vi "lateral_and_vertical_acc.vi"(4 "Aerodyn output":T3, 5 "Vehicle Param":T2, 6 "Pdyn2":T1, 7 "FE_b [N], FG [N], FA [N], Fco[N]":T4, 8 "Data":dbl[][](array[numeric]), 9 "Time":T5, 10 "acc [m/s^2]":dbl[](array[numeric]), 11 "Rotation":T6) -> (3 "k_acc":cluster{"lat_acc_mod":dbl, "up_acc":dbl})   [LabVIEW 2017]
uses:
  <vilib>/Analysis/coordinate.llb/Euler Rotation Order.ctl
  <vilib>/Analysis/_algsub.llb/Vector Norm Type.ctl
  <vilib>/Analysis/_algsub.llb/Real Vector Norm.vi
  <vilib>/Analysis/baseanly.llb/Real A x B.vi
  <vilib>/Analysis/baseanly.llb/Real Dot Product.vi
  <vilib>/Analysis/Matrix/Numeric/Conversions/Array To Matrix - RA2.vi
  <vilib>/Analysis/Matrix/Numeric/Conversions/Matrix To Array - RM.vi
  <vilib>/Analysis/Matrix/Numeric/Conversions/Array To Matrix - RA.vi
  <vilib>/Analysis/NI_AALPro.lvlib
  <vilib>/Analysis/Matrix/NI_Matrix.lvlib
  <vilib>/Analysis/NI_AALBase.lvlib
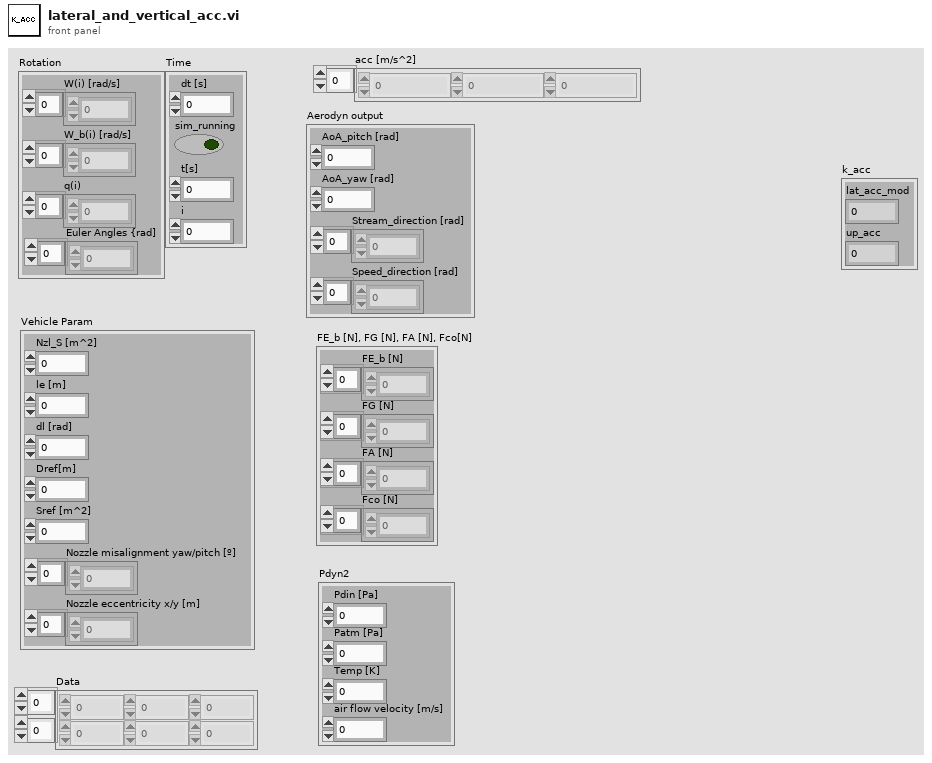
[diagram p1: front panel]
types:
  T1 = cluster{"Pdin [Pa]":dbl, "Patm [Pa]":dbl, "Temp [K]":dbl, "air flow velocity [m/s]":dbl}
  T2 = cluster{"Nzl_S [m^2]":dbl, "le [m]":dbl, "dl [rad]":dbl, "Dref[m]":dbl, "Sref [m^2]":dbl, "Nozzle misalignment yaw/pitch [º]":dbl[], "Nozzle eccentricity x/y [m]":dbl[]}
  T3 = cluster{"AoA_pitch [rad]":dbl, "AoA_yaw [rad]":dbl, "Stream_direction [rad]":dbl[], "Speed_direction [rad]":dbl[]}
  T4 = cluster{"FE_b [N]":dbl[], "FG [N]":dbl[], "FA [N]":dbl[], "Fco [N]":dbl[]}
  T5 = cluster{"dt [s]":dbl, "sim_running":bool, "t[s]":dbl, "i":i32}
  T6 = cluster{"W(i) [rad/s]":dbl[], "W_b(i) [rad/s]":dbl[], "q(i)":dbl[], "Euler Angles {rad]":dbl[]}
  T7 = typedef "NI_AALPro.lvlib/Vector Norm Type.ctl" = u16
  T8 = cluster{"AoA_pitch [rad]":dbl, "AoA_yaw [rad]":dbl, "Stream_direction [rad]":dbl[]}
  T9 = typedef "NI_AALPro.lvlib/Euler Rotation Order.ctl" = u16
  T10 = typedef "NI_Matrix.lvlib/RealMatrix.ctl" = dbl[][]
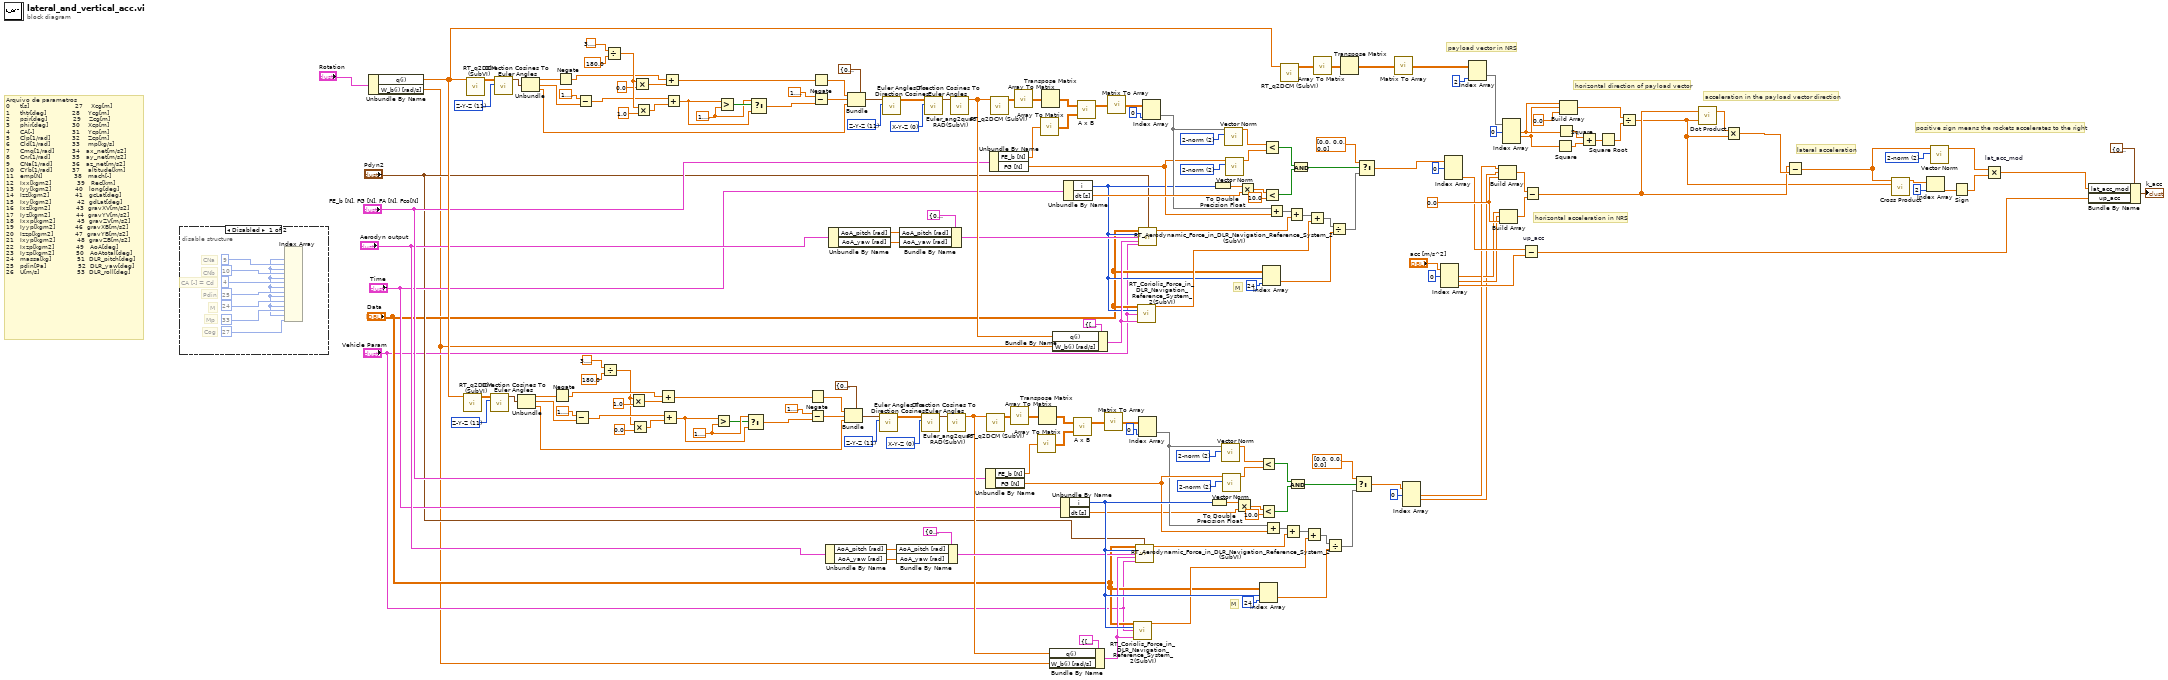
[diagram p0: block diagram]
diagram:
  w62 = T7 2 items=["1-norm"=1, "2-norm"=2, "Inf-norm"=3, "-Inf-norm"=4, "User Defined"=5] ("norm type")
  w61 = T7 2 items=["1-norm"=1, "2-norm"=2, "Inf-norm"=3, "-Inf-norm"=4, "User Defined"=5] ("norm type")
  w43 = T9 0 items=["X-Y-Z", "X-Z-Y", "Y-X-Z", "Y-Z-X", "Z-X-Y", "Z-Y-X", "X-Y-X", "X-Z-X", "Y-X-Y", "Y-Z-Y", "Z-X-Z", "Z-Y-Z"] ("rotation order")
  w42 = T9 11 items=["X-Y-Z", "X-Z-Y", "Y-X-Z", "Y-Z-X", "Z-X-Y", "Z-Y-X", "X-Y-X", "X-Z-X", "Y-X-Y", "Y-Z-Y", "Z-X-Z", "Z-Y-Z"] ("rotation order")
  w33 = 1.5707963267948966
  w17 = T9 11 items=["X-Y-Z", "X-Z-Y", "Y-X-Z", "Y-Z-X", "Z-X-Y", "Z-Y-X", "X-Y-X", "X-Z-X", "Y-X-Y", "Y-Z-Y", "Z-X-Z", "Z-Y-Z"] ("rotation order")
  w97 = T7 2 items=["1-norm"=1, "2-norm"=2, "Inf-norm"=3, "-Inf-norm"=4, "User Defined"=5] ("norm type")
  w113 = 0.0 ("element")
  w143 = T7 2 items=["1-norm"=1, "2-norm"=2, "Inf-norm"=3, "-Inf-norm"=4, "User Defined"=5] ("norm type")
  w144 = T7 2 items=["1-norm"=1, "2-norm"=2, "Inf-norm"=3, "-Inf-norm"=4, "User Defined"=5] ("norm type")
  w162 = T9 0 items=["X-Y-Z", "X-Z-Y", "Y-X-Z", "Y-Z-X", "Z-X-Y", "Z-Y-X", "X-Y-X", "X-Z-X", "Y-X-Y", "Y-Z-Y", "Z-X-Z", "Z-Y-Z"] ("rotation order")
  w163 = T9 11 items=["X-Y-Z", "X-Z-Y", "Y-X-Z", "Y-Z-X", "Z-X-Y", "Z-Y-X", "X-Y-X", "X-Z-X", "Y-X-Y", "Y-Z-Y", "Z-X-Z", "Z-Y-Z"] ("rotation order")
  w172 = 1.5707963267948966
  w188 = T9 11 items=["X-Y-Z", "X-Z-Y", "Y-X-Z", "Y-Z-X", "Z-X-Y", "Z-Y-X", "X-Y-X", "X-Z-X", "Y-X-Y", "Y-Z-Y", "Z-X-Z", "Z-Y-Z"] ("rotation order")
  # "M"
  # "positive sign means the rockets accelerates to the right"
  # "lateral acceleration"
  # "acceleration in the payload vector direction"
  # "horizontal direction of payload vector"
  # "horizontal acceleration in NRS"
  # "payload vector in NRS"
  # "M"
  # "Arquivo de parametros\n0     t[s]                       27    Xcg[m] \n1     thtr[deg]             28    Ycg[m]\n2     psir[deg]             29    Zcg[m]  \n3     phir[deg]            30    Xcp[m]       \n4     CA[-]                   31    Ycp[m]        \n5     Clp[1/rad]           32    Zcp[m]     \n6     Cld[1/rad]           33    mp[kg/s]        \n7     Cmq[1/rad]         34   ax_net[m/s2]         \n8     Cnr[1/rad]           35   ay_net[m/s2]      \n9     CNa[1/rad]          36   az_net[m/s2]      \n10   CYb[1/rad]          37    altitude[km]       \n11   emp[N]                38   mach[-]     \n12   Ixx[kgm2]             39   Rec[km]     \n13   Iyy[kgm2]            40   long[deg]     \n14   Izz[kgm2]             41   gcLat[deg]        \n15   Ixy[kgm2]             42  gdLat[deg]       \n16   Ixz[kgm2]             43  gravXV[m/s2]  \n17   Iyz[kgm2]             44  gravYV[m/s2]     \n18   Ixxp[kgm2]           45  gravZV[m/s2]         \n19   Iyyp[kgm2]          46  gravXB[m/s2]         \n20   Izzp[kgm2]           47  gravYB[m/s2]         \n21   Ixyp[kgm2]           48  gravZB[m/s2]           \n22   Ixzp[kgm2]           49   AoA[deg]             \n23   Iyzp[kgm2]           50   AoAtotal[deg]       \n24   massa[kg]             51  DLR_pitch[deg]    \n25   pdin[Pa]                52  DLR_yaw[deg]  \n26   U[m/s]                   53  DLR_roll[deg]"
  n1 = disable-structure shown="Disabled" {
    frame Disabled {
      # "Cog"
      # "Mp"
      # "M"
      # "Pdin"
      # "CA [-] = Cd"
      # "CNb"
      # "CNa"
      n2 = Index Array(index (col) #1=9 ("disabled index (col)"), index (row) #2=w191, index (col) #2=10 ("disabled index (col)"), index (row) #3=w191, index (col) #3=4 ("disabled index (col)"), index (row) #4=w191, index (col) #4=25 ("disabled index (col)"), index (row) #5=w191, index (col) #5=24 ("disabled index (col)"), index (row) #6=w191, index (col) #6=33 ("disabled index (col)"), index (row) #7=w191, index (col) #7=27 ("disabled index (col)")) -> (index (row) #1=w191:i32)  [unwired: 1 in, 7 out]
    }
    frame Enabled {
    }
  }
  n3 = Unbundle By Name("Rotation") -> ("q(i)"=w15:dbl[], "W_b(i) [rad/s]"=w8:dbl[])
  n4 = call "RT_q2DCM (SubVI).vi"("Quaternion"=w15) -> ("DCM"=w16:dbl[][])  [unwired: 10 in]
  n5 = call "RT_q2DCM (SubVI).vi"("Quaternion"=w15) -> ("DCM"=w189:dbl[][])  [unwired: 10 in]
  n6 = call <vilib>:"Direction Cosines To Euler Angles.vi"("rotation order"=w17, "Direction Cosines"=w16) -> ("Euler Angles"=w18:cluster{"phi":dbl, "theta":dbl, "psi":dbl})  [unwired: 8 in, 1 out]
  n7 = call <vilib>:"Direction Cosines To Euler Angles.vi"("rotation order"=w188, "Direction Cosines"=w189) -> ("Euler Angles"=w187:cluster{"phi":dbl, "theta":dbl, "psi":dbl})  [unwired: 8 in, 1 out]
  n8 = Unbundle(w18) -> ("phi"=w19:dbl, "theta"=w21:dbl, "psi"=w40:dbl)
  n9 = Unbundle(w187) -> ("phi"=w186:dbl, "theta"=w184:dbl, "psi"=w165:dbl)
  n10 = Negate(x=w19) -> (-x=w28:dbl)
  n11 = Negate(x=w186) -> (-x=w177:dbl)
  n12 = Subtract(x=1.5707963267948966, y=w21) -> (x-y=w30:dbl)
  n13 = Subtract(x=1.5707963267948966, y=w184) -> (x-y=w175:dbl)
  n14 = Divide(x=3.141592653589793, y=180.0) -> (x/y=w24:dbl)
  n15 = Divide(x=3.141592653589793, y=180.0) -> (x/y=w181:dbl)
  n16 = Multiply(x=w24, y=1.0) -> (x*y=w27:dbl)
  n17 = Multiply(x=w24, y=0.0) -> (x*y=w29:dbl)
  n18 = Multiply(x=w181, y=0.0) -> (x*y=w178:dbl)
  n19 = Multiply(x=w181, y=1.0) -> (x*y=w176:dbl)
  n20 = Add(x=w28, y=w27) -> (x+y=w35:dbl)
  n21 = Add(x=w30, y=w29) -> (x+y=w32:dbl)
  n22 = Add(x=w177, y=w178) -> (x+y=w170:dbl)
  n23 = Add(x=w175, y=w176) -> (x+y=w173:dbl)
  n24 = Greater?(x=w32, y=w33) -> (0:w31:bool)
  n25 = Greater?(x=w173, y=w172) -> (0:w174:bool)
  n26 = Select(t=w33, s=w31, f=w32) -> (s? t:f=w38:dbl)
  n27 = Select(t=w172, s=w174, f=w173) -> (s? t:f=w167:dbl)
  n28 = Negate(x=w35) -> (-x=w36:dbl)
  n29 = Subtract(x=1.5707963267948966, y=w38) -> (x-y=w39:dbl)
  n30 = Negate(x=w170) -> (-x=w169:dbl)
  n31 = Subtract(x=1.5707963267948966, y=w167) -> (x-y=w166:dbl)
  n32 = Unbundle By Name("Aerodyn output") -> ("AoA_pitch [rad]"=w58:dbl, "AoA_yaw [rad]"=w59:dbl)
  n33 = Unbundle By Name("Aerodyn output") -> ("AoA_pitch [rad]"=w147:dbl, "AoA_yaw [rad]"=w146:dbl)
  n34 = Bundle(cluster=cluster{"phi":dbl, "theta":dbl, "psi":dbl} {"phi"=0.0, "theta"=0.0, "psi"=0.0} ("Euler Angles"), "phi"=w36, "theta"=w39, "psi"=w40) -> (w41:cluster{"phi":dbl, "theta":dbl, "psi":dbl})
  n35 = Bundle(cluster=cluster{"phi":dbl, "theta":dbl, "psi":dbl} {"phi"=0.0, "theta"=0.0, "psi"=0.0} ("Euler Angles"), "phi"=w169, "theta"=w166, "psi"=w165) -> (w164:cluster{"phi":dbl, "theta":dbl, "psi":dbl})
  n36 = call <vilib>:"Euler Angles To Direction Cosines.vi"("rotation order"=w42, "Euler Angles"=w41) -> ("Direction Cosines"=w44:dbl[][])  [unwired: 8 in, 1 out]
  n37 = call <vilib>:"Euler Angles To Direction Cosines.vi"("rotation order"=w163, "Euler Angles"=w164) -> ("Direction Cosines"=w161:dbl[][])  [unwired: 8 in, 1 out]
  n38 = Bundle By Name(cluster=T8 {"AoA_pitch [rad]"=0.0, "AoA_yaw [rad]"=0.0, "Stream_direction [rad]"=[]} ("output cluster"), "AoA_pitch [rad]"=w58, "AoA_yaw [rad]"=w59) -> (w57:T8)
  n39 = Bundle By Name(cluster=T8 {"AoA_pitch [rad]"=0.0, "AoA_yaw [rad]"=0.0, "Stream_direction [rad]"=[]} ("output cluster"), "AoA_pitch [rad]"=w147, "AoA_yaw [rad]"=w146) -> (w148:T8)
  n40 = call <vilib>:"Direction Cosines To Euler Angles.vi"("rotation order"=w43, "Direction Cosines"=w44) -> ("Euler Angles"=w45:cluster{"phi":dbl, "theta":dbl, "psi":dbl})  [unwired: 8 in, 1 out]
  n41 = call <vilib>:"Direction Cosines To Euler Angles.vi"("rotation order"=w162, "Direction Cosines"=w161) -> ("Euler Angles"=w160:cluster{"phi":dbl, "theta":dbl, "psi":dbl})  [unwired: 8 in, 1 out]
  n42 = call "Euler_ang2quat RAD(SubVI).vi"("Euler Angles [rad]"=w45) -> ("Quaternions"=w55:dbl[])  [unwired: 10 in]
  n43 = call "Euler_ang2quat RAD(SubVI).vi"("Euler Angles [rad]"=w160) -> ("Quaternions"=w150:dbl[])  [unwired: 10 in]
  n44 = Unbundle By Name("FE_b [N], FG [N], FA [N], Fco[N]") -> ("FE_b [N]"=w50:dbl[], "FG [N]"=w76:dbl[])
  n45 = call "RT_q2DCM (SubVI).vi"("Quaternion"=w55) -> ("DCM"=w46:dbl[][])  [unwired: 10 in]
  n46 = Unbundle By Name("FE_b [N], FG [N], FA [N], Fco[N]") -> ("FE_b [N]"=w155:dbl[], "FG [N]"=w129:dbl[])
  n47 = call "RT_q2DCM (SubVI).vi"("Quaternion"=w150) -> ("DCM"=w159:dbl[][])  [unwired: 10 in]
  n48 = call-poly <vilib>:"Array To Matrix.vi"("Real 2D Array"=w46) -> ("Real Matrix"=w47:T10)
  n49 = call-poly <vilib>:"Array To Matrix.vi"("Real 2D Array"=w159) -> ("Real Matrix"=w158:T10)
  n50 = call-poly <vilib>:"Array To Matrix.vi"("Real 1D Array"=w50) -> ("Real Matrix (Column Vector)"=w49:T10)
  n51 = Transpose Matrix(1:w47) -> (0:w48:T10)
  n52 = call-poly <vilib>:"Array To Matrix.vi"("Real 1D Array"=w155) -> ("Real Matrix (Column Vector)"=w156:T10)
  n53 = Transpose Matrix(1:w158) -> (0:w157:T10)
  n54 = Bundle By Name(cluster=T6 {"W(i) [rad/s]"=[], "W_b(i) [rad/s]"=[], "q(i)"=[], "Euler Angles {rad]"=[]} ("Rotation 2"), "q(i)"=w55, "W_b(i) [rad/s]"=w8) -> (w60:T6)
  n55 = Bundle By Name(cluster=T6 {"W(i) [rad/s]"=[], "W_b(i) [rad/s]"=[], "q(i)"=[], "Euler Angles {rad]"=[]} ("Rotation 2"), "q(i)"=w150, "W_b(i) [rad/s]"=w8) -> (w145:T6)
  n56 = Unbundle By Name("Time") -> ("i"=w79:i32, "dt [s]"=w65:dbl)
  n57 = Unbundle By Name("Time") -> ("i"=w126:i32, "dt [s]"=w140:dbl)
  n58 = call-poly <vilib>:"A x B.vi"("B"=w49, "A"=w48) -> ("A x B"=w53:T10)  [unwired: 1 out]
  n59 = call-poly <vilib>:"A x B.vi"("B"=w156, "A"=w157) -> ("A x B"=w152:T10)  [unwired: 1 out]
  n60 = call-poly <vilib>:"Matrix To Array.vi"("Real Matrix"=w53) -> ("Real 2D Array"=w51:dbl[][])
  n61 = call-poly <vilib>:"Matrix To Array.vi"("Real Matrix"=w152) -> ("Real 2D Array"=w154:dbl[][])
  n62 = call "RT_Coriolis_Force_in_DLR_Navigation_Reference_System_2(SubVI).vi"("Data"="Data", "i"=w79, "Vehicle Parameters"="Vehicle Param", "Rotation"=w60) -> ("Fco (N)"=w78:dbl[])  [unwired: 11 in]
  n63 = call "RT_Aerodynamic_Force_in_DLR_Navigation_Reference_System_2 (SubVI).vi"("Data"="Data", "input cluster 3"="Pdyn2", "i"=w79, "output cluster"=w57, "Rotation"=w60, "Vehicle Parameters"="Vehicle Param") -> ("FA"=w77:dbl[])  [unwired: 8 in, 1 out]
  n64 = call "RT_Coriolis_Force_in_DLR_Navigation_Reference_System_2(SubVI).vi"("Data"="Data", "i"=w126, "Vehicle Parameters"="Vehicle Param", "Rotation"=w145) -> ("Fco (N)"=w127:dbl[])  [unwired: 11 in]
  n65 = call "RT_Aerodynamic_Force_in_DLR_Navigation_Reference_System_2 (SubVI).vi"("Data"="Data", "input cluster 3"="Pdyn2", "i"=w126, "output cluster"=w148, "Rotation"=w145, "Vehicle Parameters"="Vehicle Param") -> ("FA"=w128:dbl[])  [unwired: 8 in, 1 out]
  n66 = Index Array(array=w51, index (col)=0 ("index (row)")) -> (element=w75:dbl[])  [unwired: 1 in]
  n67 = Index Array(array=w154, index (col)=0 ("index (row)")) -> (element=w130:dbl[])  [unwired: 1 in]
  n68 = To Double Precision Float(number=w79) -> (double precision float=w66:dbl)
  n69 = To Double Precision Float(number=w126) -> (double precision float=w139:dbl)
  n70 = call-poly <vilib>:"Vector Norm.vi"("norm type"=w61, "Input Vector"=w75) -> ("norm"=w63:dbl)  [unwired: 8 in, 1 out]
  n71 = call-poly <vilib>:"Vector Norm.vi"("norm type"=w62, "Input Vector"=w76) -> ("norm"=w64:dbl)  [unwired: 8 in, 1 out]
  n72 = call-poly <vilib>:"Vector Norm.vi"("norm type"=w144, "Input Vector"=w130) -> ("norm"=w142:dbl)  [unwired: 8 in, 1 out]
  n73 = call-poly <vilib>:"Vector Norm.vi"("norm type"=w143, "Input Vector"=w129) -> ("norm"=w141:dbl)  [unwired: 8 in, 1 out]
  n74 = Multiply(x=w66, y=w65) -> (x*y=w67:dbl)
  n75 = Multiply(x=w139, y=w140) -> (x*y=w138:dbl)
  n76 = Index Array(array="Data", index (row)=w79, index (col)=24 ("disabled index (col)")) -> (element=w82:dbl)
  n77 = Less?(x=w63, y=w64) -> (x < y?=w69:bool)
  n78 = Less?(x=w67, y=10.0) -> (x < y?=w70:bool)
  n79 = Index Array(array="Data", index (row)=w126, index (col)=24 ("disabled index (col)")) -> (element=w123:dbl)
  n80 = Less?(x=w142, y=w141) -> (x < y?=w136:bool)
  n81 = Less?(x=w138, y=10.0) -> (x < y?=w135:bool)
  n82 = Add(x=w75, y=w76) -> (x+y=w73:dbl[])
  n83 = Add(x=w130, y=w129) -> (x+y=w132:dbl[])
  n84 = call "RT_q2DCM (SubVI).vi"("Quaternion"=w15) -> ("DCM"=w120:dbl[][])  [unwired: 10 in]
  n85 = Add(x=w73, y=w77) -> (x+y=w74:dbl[])
  n86 = Add(x=w132, y=w128) -> (x+y=w131:dbl[])
  n87 = And(x=w69, y=w70) -> (x .and. y?=w71:bool)
  n88 = And(x=w136, y=w135) -> (x .and. y?=w134:bool)
  n89 = Add(x=w74, y=w78) -> (x+y=w81:dbl[])
  n90 = Add(x=w131, y=w127) -> (x+y=w124:dbl[])
  n91 = call-poly <vilib>:"Array To Matrix.vi"("Real 2D Array"=w120) -> ("Real Matrix"=w121:T10)
  n92 = Divide(x=w81, y=w82) -> (x/y=w83:dbl[])
  n93 = Divide(x=w124, y=w123) -> (x/y=w122:dbl[])
  n94 = Transpose Matrix(1:w121) -> (0:w117:T10)
  n95 = Select(t=dbl[] [0.0, 0.0, 0.0], s=w71, f=w83) -> (s? t:f=w2:dbl[])
  n96 = Select(t=dbl[] [0.0, 0.0, 0.0], s=w134, f=w122) -> (s? t:f=w84:dbl[])
  n97 = call-poly <vilib>:"Matrix To Array.vi"("Real Matrix"=w117) -> ("Real 2D Array"=w118:dbl[][])
  n98 = Index Array(array=w2, index #1=0 ("index")) -> (element #1=w6:dbl, element #2=w3:dbl)  [unwired: 2 in, 1 out]
  n99 = Index Array(array="acc [m/s^2]", index #1=0 ("index")) -> (element #1=w5:dbl, element #2=w4:dbl, element #3=w89:dbl)  [unwired: 2 in]
  n100 = Index Array(array=w84, index #1=0 ("index")) -> (element #3=w90:dbl)  [unwired: 2 in, 2 out]
  n101 = Index Array(array=w118, index (col)=2 ("index (row)")) -> (element=w109:dbl[])  [unwired: 1 in]
  n102 = Build Array(w6, w3, w113) -> (w112:dbl[])
  n103 = Build Array(w5, w4, w113) -> (w111:dbl[])
  n104 = Index Array(array=w109, index #1=0 ("index")) -> (element #1=w105:dbl, element #2=w104:dbl)  [unwired: 2 in, 1 out]
  n105 = Subtract "up_acc"(x=w90, y=w89) -> (x-y=w86:dbl)
  n106 = Subtract(x=w112, y=w111) -> (x-y=w98:dbl[])
  n107 = Square(x=w104) -> (x^2=w108:dbl)
  n108 = Square(x=w105) -> (x^2=w106:dbl)
  n109 = Build Array(w105, w104, 0.0 ("element")) -> (w102:dbl[])
  n110 = Add(x=w106, y=w108) -> (x+y=w107:dbl)
  n111 = Square Root(x=w107) -> (sqrt(x)=w101:dbl)
  n112 = Divide(x=w102, y=w101) -> (x/y=w1:dbl[])
  n113 = call-poly <vilib>:"Dot Product.vi"("Y Vector"=w1, "X Vector"=w98) -> ("X * Y"=w100:dbl)  [unwired: 1 out]
  n114 = Multiply(x=w100, y=w1) -> (x*y=w99:dbl[])
  n115 = Subtract(x=w98, y=w99) -> (x-y=w96:dbl[])
  n116 = call <vilib>:"Cross Product.vi"("B Vector"=w1, "A Vector"=w96) -> ("Cross Product"=w95:dbl[])  [unwired: 8 in, 1 out]
  n117 = Index Array(array=w95, index=2) -> (element=w93:dbl)
  n118 = call-poly <vilib>:"Vector Norm.vi"("norm type"=w97, "Input Vector"=w96) -> ("norm"=w92:dbl)  [unwired: 8 in, 1 out]
  n119 = Sign(1:w93) -> (0:w91:dbl)
  n120 = Multiply "lat_acc_mod"(x=w92, y=w91) -> (x*y=w85:dbl)
  n121 = Bundle By Name(cluster=cluster{"lat_acc_mod":dbl, "up_acc":dbl} {"lat_acc_mod"=0.0, "up_acc"=0.0} ("k_acc 2"), "lat_acc_mod"=w85, "up_acc"=w86) -> (→"k_acc":cluster{"lat_acc_mod":dbl, "up_acc":dbl})
